vi "Basic SyRen 50 Controller_VarSpeed.vi"() -> ()   [LabVIEW 2016]
uses:
  <vilib>/Instr/_visa.llb/VISA Configure Serial Port (Instr).vi
panel:
  in  "Speed/Direction":u8(slide)=128 scale=0.0..255.0
  in  "baud rate (9600)":u32=38400
  in  "VISA resource name":refnum<visa-resource-name>="COM1"
  out "error out":errorcluster
  in  "Stop Button":bool
  in  "error in":errorcluster
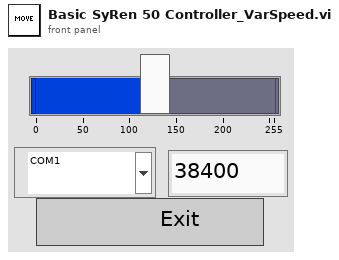
[diagram p1: front panel]
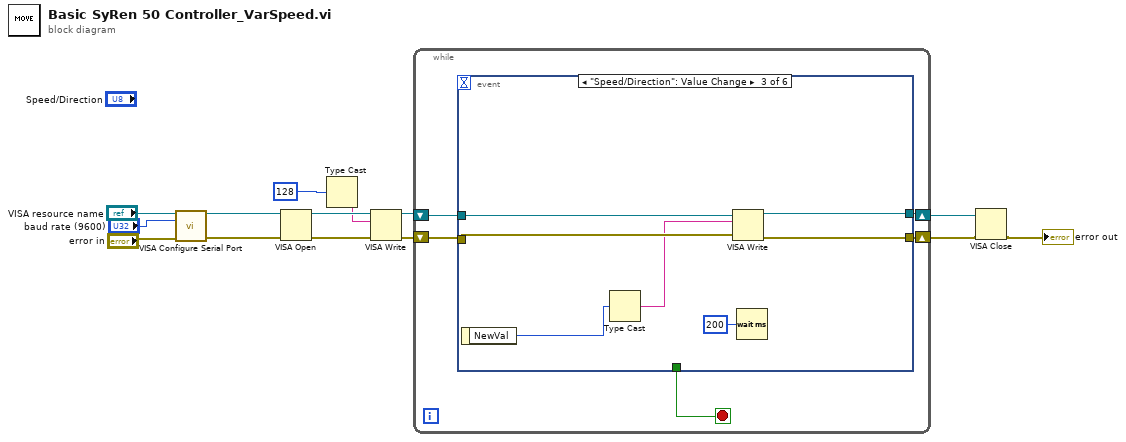
[diagram p0: block diagram]
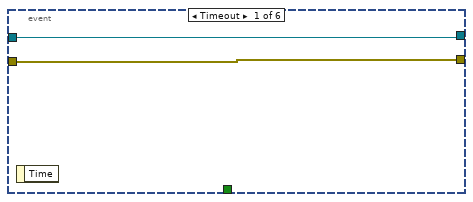
[diagram p2: hidden frame]
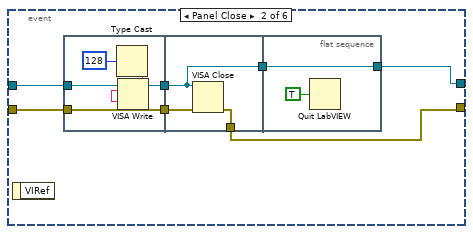
[diagram p3: hidden frame]
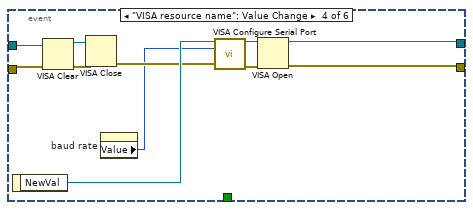
[diagram p4: hidden frame]
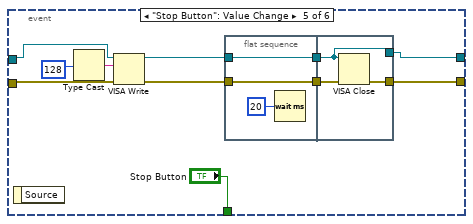
[diagram p5: hidden frame]
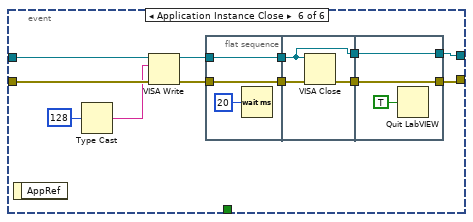
[diagram p6: hidden frame]
diagram:
  n1 = call-poly "VISA Configure Serial Port"("VISA resource name"="VISA resource name", "baud rate (9600)"="baud rate (9600)", "error in (no error)"="error in") -> ("VISA resource name out"=w12:refnum<visa-resource-name>, "error out"=w11:errorcluster)  [unwired: 11 in]
  n2 = VISA Open(error in (no error)=w11, VISA resource name=w12) -> (VISA resource name=w7:refnum<visa-resource-name>, error out=w8:errorcluster)  [unwired: 3 in]
  n3 = Type Cast(x=u8 128 ("Speed & Direction")) -> (*(type *) &x=w5:string)  [unwired: 1 in]
  n4 = VISA Write(VISA resource name=w7, write buffer=w5, error in (no error)=w8) -> (VISA resource name out=w4:refnum<visa-resource-name>, error out=w6:errorcluster)  [unwired: 1 out]
  n5 = while {
    shift-right: [w15] -> w1
    shift-left: w4 -> [w16]
    shift-right: [w18] -> w3
    shift-left: w6 -> [w19]
    stop <- w17 stop-if-true
    n6 = event shown="[2] \"Speed/Direction\": Value Change" {
      selector: _ -> [_ _ _ _ _ _]
      dyn-events: _ -> [_ _ _ _ _ _]
      timeout: _ -> [_ _ _ _ _ _]
      tunnel: w19 -> [w21 w28 w44 w53 w62 w80]
      tunnel: [w21 w24 w45 w47 w65 w85] -> w18
      tunnel: [_ _ _ _ "Stop Button" _] -> w17
      tunnel: w16 -> [w20 w26 w42 w54 w59 w78]
      tunnel: [w20 w23 w43 w46 w57 w75] -> w15
      event Timeout {
        n7 = event-data() -> ()  [unwired: 1 in, 1 out]
      }
      event Panel Close {
        n8 = event-data() -> ()  [unwired: 1 in, 1 out]
        n9 = flat-sequence {
          tunnel: w28 -> [w33]
          tunnel: [w33] -> w27
          tunnel: w26 -> [w31]
          tunnel: [w29] -> w25
          tunnel: w27 -> [w36]
          tunnel: w25 -> [w34]
          tunnel: [w35] -> w24
          tunnel: [w34] -> w22
          tunnel: [w37] -> w23
          tunnel: w22 -> [w37]
          frame #0 {
            n10 = Type Cast(x=i16 128 ("Speed & Direction")) -> (*(type *) &x=w30:string)  [unwired: 1 in]
            n11 = VISA Write(VISA resource name=w31, write buffer=w30) -> (VISA resource name out=w29:refnum<visa-resource-name>)  [unwired: 1 in, 2 out]
          }
          frame #1 {
            n12 = VISA Close(VISA resource name=w34, error in (no error)=w36) -> (error out=w35:errorcluster)
          }
          frame #2 {
            n13 = Quit LabVIEW(quit? (T)=TRUE) -> ()
          }
        }
      }
      event "Speed/Direction": Value Change {
        n14 = event-data() -> ("NewVal"=w39:u8)  [unwired: 1 in]
        n15 = Type Cast(x=w39) -> (*(type *) &x=w40:string)  [unwired: 1 in]
        n16 = VISA Write(VISA resource name=w42, write buffer=w40, error in (no error)=w44) -> (VISA resource name out=w43:refnum<visa-resource-name>, error out=w45:errorcluster)  [unwired: 1 out]
        n17 = Wait (ms)(milliseconds to wait=u32 200) -> ()  [unwired: 1 out]
      }
      event "VISA resource name": Value Change {
        n18 = event-data() -> ("NewVal"=w50:refnum<visa-resource-name>)  [unwired: 1 in]
        n19 = VISA Clear(VISA resource name=w54, error in (no error)=w53) -> (VISA resource name out=w55:refnum<visa-resource-name>, error out=w56:errorcluster)
        n20 = VISA Close(VISA resource name=w55, error in (no error)=w56) -> (error out=w49:errorcluster)
        n21 = property on="baud rate" class="DigNum (strict)"() -> ("Value"=w48:u32)  [unwired: 2 in, 2 out]
        n22 = call-poly "VISA Configure Serial Port"("VISA resource name"=w50, "baud rate (9600)"=w48, "error in (no error)"=w49) -> ("VISA resource name out"=w51:refnum<visa-resource-name>, "error out"=w52:errorcluster)  [unwired: 11 in]
        n23 = VISA Open(error in (no error)=w52, VISA resource name=w51) -> (VISA resource name=w46:refnum<visa-resource-name>, error out=w47:errorcluster)  [unwired: 3 in]
      }
      event "Stop Button": Value Change {
        n24 = event-data() -> ()  [unwired: 1 in, 1 out]
        n25 = Type Cast(x=i16 128 ("Speed & Direction")) -> (*(type *) &x=w60:string)  [unwired: 1 in]
        n26 = VISA Write(VISA resource name=w59, write buffer=w60, error in (no error)=w62) -> (VISA resource name out=w58:refnum<visa-resource-name>, error out=w61:errorcluster)  [unwired: 1 out]
        n27 = flat-sequence {
          tunnel: w61 -> [w69]
          tunnel: w58 -> [w70]
          tunnel: [w70] -> w64
          tunnel: [w69] -> w63
          tunnel: [w72] -> w65
          tunnel: w64 -> [w71]
          tunnel: w63 -> [w73]
          tunnel: [w71] -> w57
          frame #0 {
            n28 = Wait (ms)(milliseconds to wait=u32 20) -> ()  [unwired: 1 out]
          }
          frame #1 {
            n29 = VISA Close(VISA resource name=w71, error in (no error)=w73) -> (error out=w72:errorcluster)
          }
        }
      }
      event Application Instance Close {
        n30 = event-data() -> ()  [unwired: 1 in, 1 out]
        n31 = Type Cast(x=i16 128 ("Speed & Direction")) -> (*(type *) &x=w76:string)  [unwired: 1 in]
        n32 = VISA Write(VISA resource name=w78, write buffer=w76, error in (no error)=w80) -> (VISA resource name out=w77:refnum<visa-resource-name>, error out=w79:errorcluster)  [unwired: 1 out]
        n33 = flat-sequence {
          tunnel: w79 -> [w87]
          tunnel: w77 -> [w88]
          tunnel: [w88] -> w83
          tunnel: [w87] -> w82
          tunnel: w83 -> [w89]
          tunnel: w82 -> [w91]
          tunnel: [w90] -> w81
          tunnel: [w89] -> w74
          tunnel: [w94] -> w85
          tunnel: w81 -> [w94]
          tunnel: [w92] -> w75
          tunnel: w74 -> [w92]
          frame #0 {
            n34 = Wait (ms)(milliseconds to wait=u32 20) -> ()  [unwired: 1 out]
          }
          frame #1 {
            n35 = VISA Close(VISA resource name=w89, error in (no error)=w91) -> (error out=w90:errorcluster)
          }
          frame #2 {
            n36 = Quit LabVIEW(quit? (T)=TRUE) -> ()
          }
        }
      }
    }
  }
  n37 = VISA Close(VISA resource name=w1, error in (no error)=w3) -> (error out=→"error out":errorcluster)
